vi "remoteFocussingConversion.vi"(2 "units":u16(ring) items=["fractional", "voltage (V)", "position (um)"], 3 "mode":u16(ring) items=["direct", "inverse"], 4 "dz array":dbl[](array[numeric]), 5 "dz":dbl) -> (0 "dz array out":dbl[](array[numeric]), 1 "dz out":dbl)   [LabVIEW 2017]
uses:
  globalDevices.vi
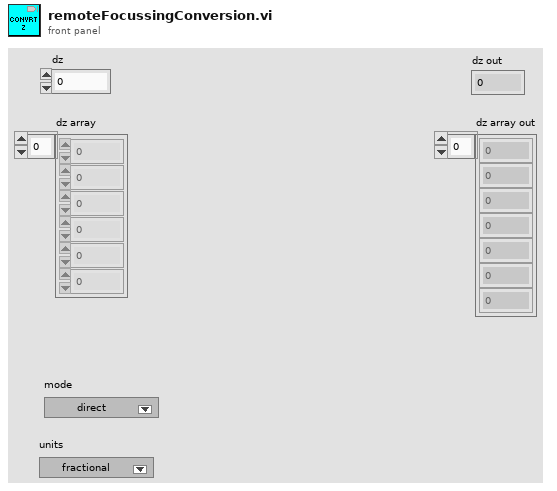
[diagram p1: front panel]
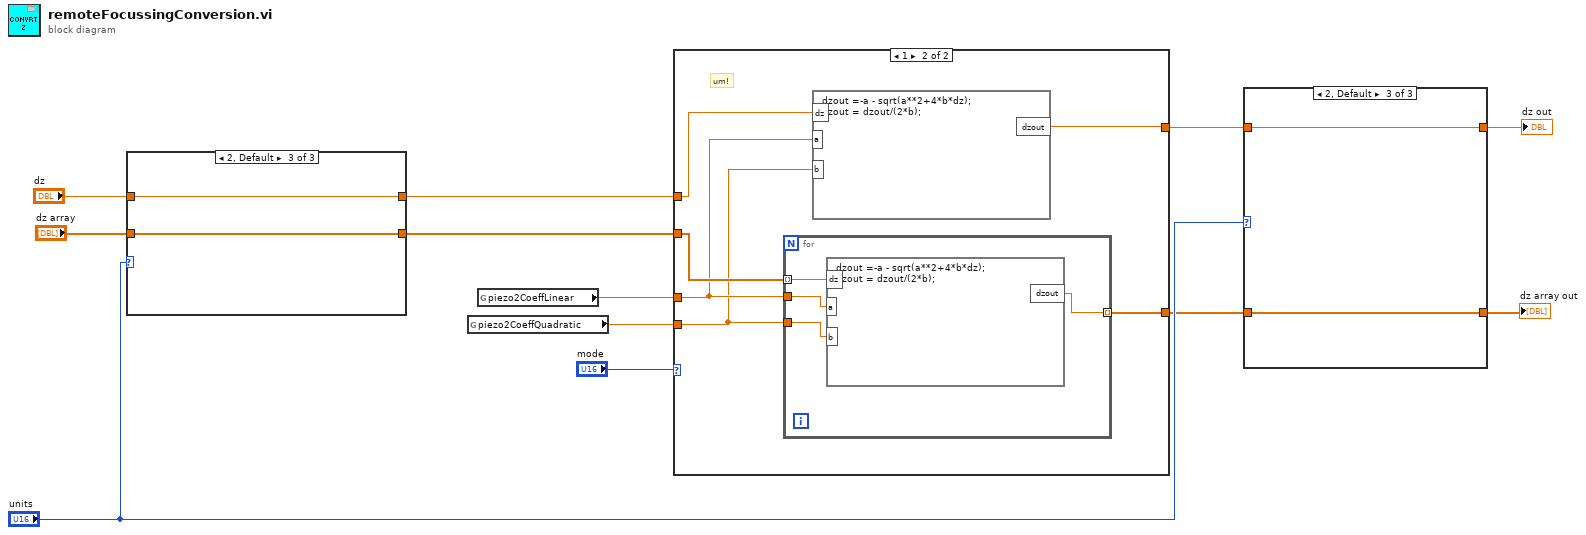
[diagram p0: block diagram]
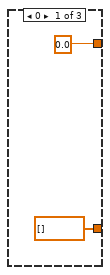
[diagram p2: hidden frame]
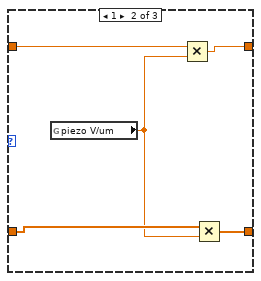
[diagram p3: hidden frame]
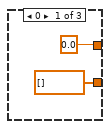
[diagram p4: hidden frame]
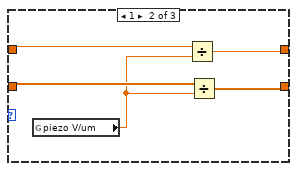
[diagram p5: hidden frame]
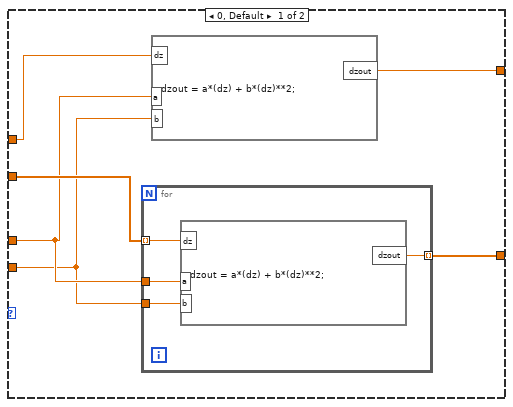
[diagram p6: hidden frame]
diagram:
  n1 = case shown="2, Default" "units" {
    tunnel: "dz" -> [_ w19 w21]
    tunnel: "dz array" -> [_ w18 w20]
    tunnel: [0.0 w16 w21] -> w7
    tunnel: [dbl[] [] ("dz array") w15 w20] -> w6
    frame 0 {
    }
    frame 1 {
      n2 = global read "globalDevices.vi" "piezo V/um"() -> (w17:dbl)
      n3 = Divide(x=w19, y=w17) -> (x/y=w16:dbl)
      n4 = Divide(x=w18, y=w17) -> (x/y=w15:dbl[])
    }
    frame 2, Default {
    }
  }
  n5 = global read "globalDevices.vi" "piezo2CoeffQuadratic"() -> (w10:dbl)
  n6 = global read "globalDevices.vi" "piezo2CoeffLinear"() -> (w11:dbl)
  n7 = case shown="1" "mode" {
    tunnel: w11 -> [w24 w34]
    tunnel: w10 -> [w23 w33]
    tunnel: w7 -> [w27 w37]
    tunnel: w6 -> [w25 w35]
    tunnel: [w26 w36] -> w3
    tunnel: [w22 w32] -> w4
    frame 0, Default {
      n8 = for {
        tunnel: w25 -> [w31] mode=indexing
        tunnel: w24 -> [w30]
        tunnel: w23 -> [w29]
        tunnel: [w28] -> w22 mode=indexing
        n9 = formula code="dzout = a*(dz) + b*(dz)**2;"("dz"=w31, "a"=w30, "b"=w29) -> ("dzout"=w28:dbl)
      }
      n10 = formula code="dzout = a*(dz) + b*(dz)**2;"("dz"=w27, "a"=w24, "b"=w23) -> ("dzout"=w26:dbl)
    }
    frame 1 {
      # "um!"
      n11 = for {
        tunnel: w35 -> [w41] mode=indexing
        tunnel: w34 -> [w40]
        tunnel: w33 -> [w39]
        tunnel: [w38] -> w32 mode=indexing
        n12 = formula code="dzout =-a - sqrt(a**2+4*b*dz);\ndzout = dzout/(2*b);"("dz"=w41, "a"=w40, "b"=w39) -> ("dzout"=w38:dbl)
      }
      n13 = formula code="dzout =-a - sqrt(a**2+4*b*dz);\ndzout = dzout/(2*b);"("dz"=w37, "a"=w34, "b"=w33) -> ("dzout"=w36:dbl)
    }
  }
  n14 = case shown="2, Default" "units" {
    tunnel: w4 -> [_ w46 w49]
    tunnel: w3 -> [_ w48 w50]
    tunnel: [0.0 w47 w50] -> w2
    tunnel: [dbl[] [] w44 w49] -> w1
    frame 0 {
    }
    frame 1 {
      n15 = global read "globalDevices.vi" "piezo V/um"() -> (w45:dbl)
      n16 = Multiply(x=w48, y=w45) -> (x*y=w47:dbl)
      n17 = Multiply(x=w46, y=w45) -> (x*y=w44:dbl[])
    }
    frame 2, Default {
    }
  }
  "dz out" <- w2
  "dz array out" <- w1
